vi "readTestDescription.vi"(8 "error in (no error)":errorcluster, 11 "Prueba in":refnum<class "Prueba.lvclass">) -> (0 "error out":errorcluster, 2 "Test Description":string="2. Ruido Intrínseco. IEC 61672-3: 2006 Cláusula 10", 3 "Prueba out":refnum<class "Prueba.lvclass">)   [LabVIEW 2019, in "Prueba.lvclass"]
uses:
  Prueba.lvclass
  Prueba.lvclass/Prueba.ctl
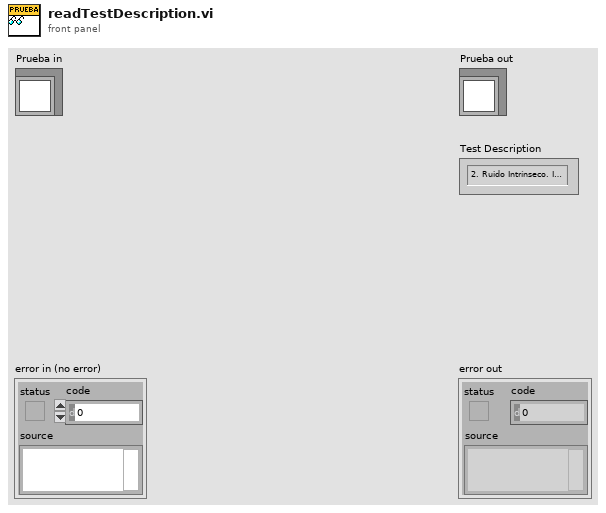
[diagram p1: front panel]
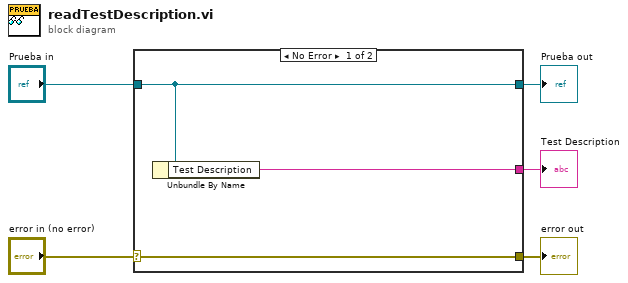
[diagram p0: block diagram]
diagram:
  n1 = case shown="No Error" "error in (no error)" {
    selector: "error in (no error)" -> [w8 w9]
    tunnel: [w8 w9] -> w4
    tunnel: [w7 w10] -> w2
    tunnel: "Prueba in" -> [w7 w10]
    tunnel: [w6 _] -> w1
    frame No Error {
      n2 = Unbundle By Name(w7) -> ("Test Description"=w6:string)
    }
    frame Error {
    }
  }
  "error out" <- w4
  "Prueba out" <- w2
  "Test Description" <- w1
